vi "Main_Mover4_Control.vi"(4 "Z (m)":dbl, 6 "Y (m)":dbl, 7 "current joint positions in":dbl[](array[numeric]), 9 "X (m)":dbl, 10 "Range acceptable?":bool, 11 "NI_Robotics_6R Type 1 Serial Arm Class in":refnum<class "NI_Robotics_6R Type 1 Serial Arm Class.lvclass">) -> (1 "Position not reachable?":bool, 2 "Simulation":refnum<vi>(3d-picture), 3 "current joint positions degree":dbl[](array[numeric]), 5 "current joint positions out":dbl[](array[numeric]))   [LabVIEW 2015]
uses:
  <vilib>/robotics/Kinematics/Analytical/6R/Type 1/NI_Robotics_6R Type 1 Serial Arm Class.lvclass
  <vilib>/robotics/Kinematics/Analytical/6R/Type 1/Analytical Inverse Kinematics (6R Type 1).vi
  <vilib>/robotics/Kinematics/NI_Kinematics.lvlib
  <vilib>/robotics/Kinematics/Analytical/NI_Robotics_AnalyticKinematics.lvlib
  <vilib>/robotics/Kinematics/Plotting/NI_Robotics_3DKinematics.lvlib
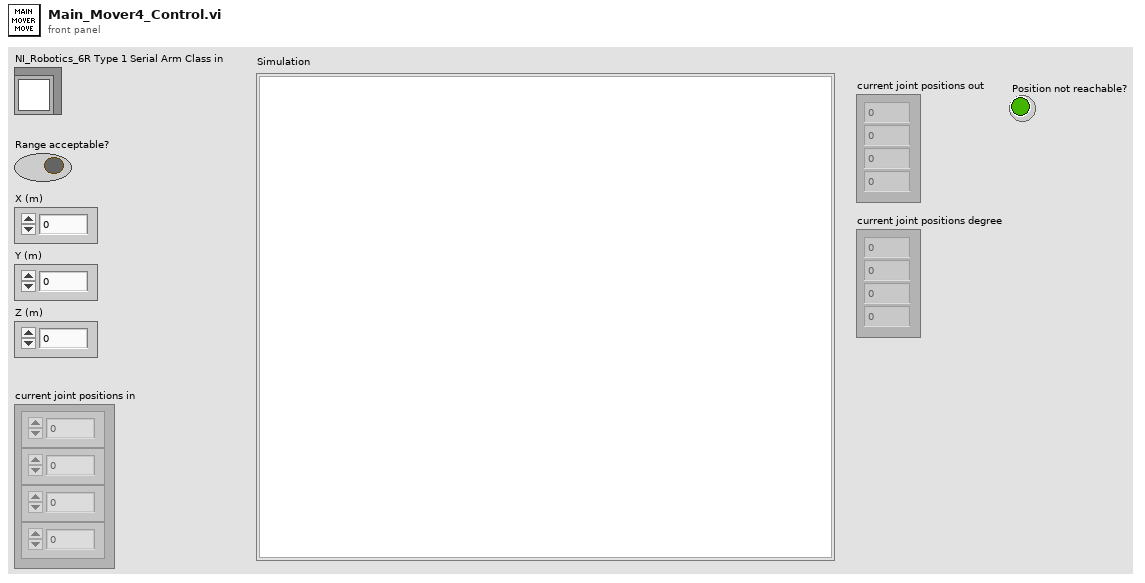
[diagram p1: front panel]
types:
  T1 = typedef "NI_Matrix.lvlib/RealMatrix.ctl" = dbl[][]
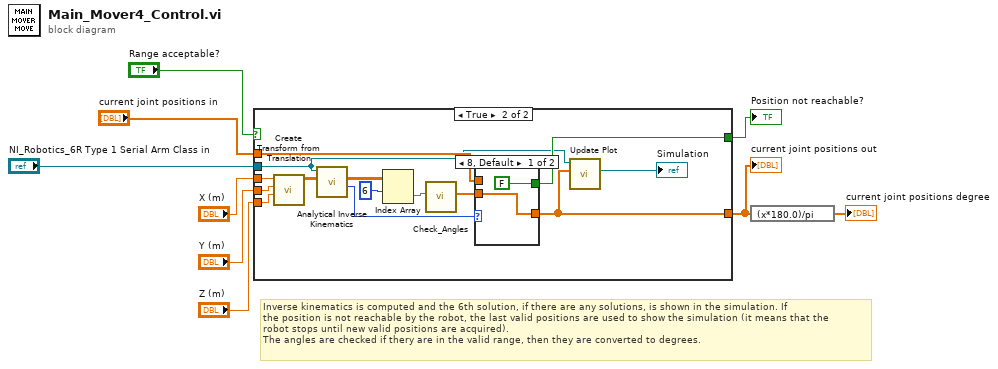
[diagram p0: block diagram]
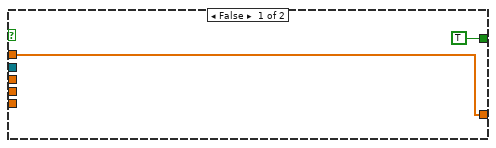
[diagram p2: hidden frame]
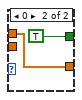
[diagram p3: hidden frame]
diagram:
  # "Inverse kinematics is computed and the 6th solution, if there are any solutions, is shown in the simulation. If\nthe position is not reachable by the robot, the last valid positions are used to show the simulation (it means that the\nrobot stops until new valid positions are acquired).\nThe angles are checked if thery are in the valid range, then they are converted to degrees."
  n1 = case shown="True" "Range acceptable?" {
    tunnel: [w11 w21] -> w6
    tunnel: [TRUE w25] -> w3
    tunnel: "current joint positions in" -> [w11 w24]
    tunnel: "NI_Robotics_6R Type 1 Serial Arm Class in" -> [_ w12]
    tunnel: "X (m)" -> [_ w15]
    tunnel: "Y (m)" -> [_ w14]
    tunnel: "Z (m)" -> [_ w13]
    frame False {
    }
    frame True {
      n2 = call <vilib>:"Create Transform from Translation.vi"("z"=w13, "y"=w14, "x"=w15) -> ("transform"=w23:T1)  [unwired: 8 in]
      n3 = call-poly <vilib>:"Analytical Inverse Kinematics.vi"("end effector transform"=w23, "6R type 1 serial arm in"=w12) -> ("number of valid solutions"=w16:i32, "joint positions"=w20:T1)  [unwired: 6 in, 2 out]
      n4 = Index Array(array=w20, index (row)=6 ("Choose solution")) -> (element=w18:dbl[])  [unwired: 1 in]
      n5 = call "Check_Angles.vi"("Joint positions (rad)"=w18) -> ("Adjusted joint positions (rad)"=w17:dbl[])  [unwired: 10 in]
      n6 = case shown="8, Default" w16 {
        tunnel: [w26 w28] -> w21
        tunnel: [FALSE TRUE] -> w25
        tunnel: w24 -> [_ w28]
        tunnel: w17 -> [w26 _]
        frame 8, Default {
        }
        frame 0 {
        }
      }
      n7 = call <vilib>:"Update Plot.vi"("joint positions"=w21, "serial arm in"=w12) -> ("serial arm scene"=→"Simulation":refnum<vi>)  [unwired: 7 in, 2 out]
    }
  }
  "current joint positions out" <- w6
  "Position not reachable?" <- w3
  n8 = expression code="(x*180.0)/pi"(w6) -> (→"current joint positions degree":dbl[])
